vi "SetRun.vi"(1 "Boolean":bool, 2 "DNet ID Number":dbl) -> ()   [LabVIEW 2011]
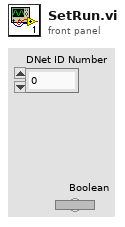
[diagram p1: front panel]
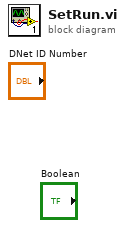
[diagram p0: block diagram]
diagram:
